vi "MACBIN Create Header__ogtk.vi"(0 "data file":path, 1 "resource file":path, 3 "error in (no error)":errorcluster) -> (4 "comment":string, 5 "header":u8[](array[numeric]), 6 "res size":i32, 7 "data refnum":refnum<file>, 8 "res refnum":refnum<file>, 9 "data size":i32, 10 "error out":errorcluster)   [LabVIEW 2018]
uses:
  <userlib>/_OpenG.lib/lvzip/macbin.llb/MACBIN Macbinary Header__ogtk.ctl
panel:
  in  "macbinary header":T1 {"last mod" format="%<%I:%M:%S %p\n%d/%m/%y>T"; "creation date" format="%<%H:%M:%S\n%d/%m/%y>T"}
  # "Please visit http://www.OpenG.org to learn about the\nOpen Source LabVIEW software movement.\n\nNOTICE -- YOU MUST LEAVE THIS NOTICE IN PLACE.  PER THE TERMS OF THE LICENSE BELOW, YOU MAY SUBLICENSE THIS SOFTWARE \nIN ANY WAY THAT DOES NOT CONFLICT WITH THIS LICENSE.\n\n### BSD License (http://www.opensource.org/licenses/bsd-license.php) Begin ###\n \nCopyright (C) 2002 Christophe Salzmann christophe.salzmann@epfl.ch\nCopyright (C) 2002 Rolf Kalbermatter rolf.kalbermatter@citengineering.com\n\nAll rights reserved.\n\nRedistribution and use in source and binary forms, with or without modification, are permitted provided that the following conditions are met:\n\n    * Redistributions of source code must retain the above copyright notice, this list of conditions and the following disclaimer.\n    * Redistributions in binary form must reproduce the above copyright notice, this list of conditions and the following disclaimer in the \n       documentation and/or other materials provided with the distribution.\n    * Neither the name of SciWare, James Kring, Inc., nor the names of its contributors may be used to endorse or promote products derived \n       from this software without specific prior written permission.\n\nTHIS SOFTWARE IS PROVIDED BY THE COPYRIGHT HOLDERS AND CONTRIBUTORS \"AS IS\" AND ANY EXPRESS OR IMPLIED WARRANTIES, \nINCLUDING, BUT NOT LIMITED TO, THE IMPLIED WARRANTIES OF MERCHANTABILITY AND FITNESS FOR A PARTICULAR PURPOSE ARE \nDISCLAIMED. IN NO EVENT SHALL THE COPYRIGHT OWNER OR CONTRIBUTORS BE LIABLE FOR ANY DIRECT, INDIRECT, INCIDENTAL,\n SPECIAL, EXEMPLARY, OR CONSEQUENTIAL DAMAGES (INCLUDING, BUT NOT LIMITED TO, PROCUREMENT OF SUBSTITUTE GOODS OR \nSERVICES; LOSS OF USE, DATA, OR PROFITS; OR BUSINESS INTERRUPTION) HOWEVER CAUSED AND ON ANY THEORY OF LIABILITY, \nWHETHER IN CONTRACT, STRICT LIABILITY, OR TORT (INCLUDING NEGLIGENCE OR OTHERWISE) ARISING IN ANY WAY OUT OF THE USE \nOF THIS SOFTWARE, EVEN IF ADVISED OF THE POSSIBILITY OF SUCH DAMAGE.\n\n### BSD License End ###"
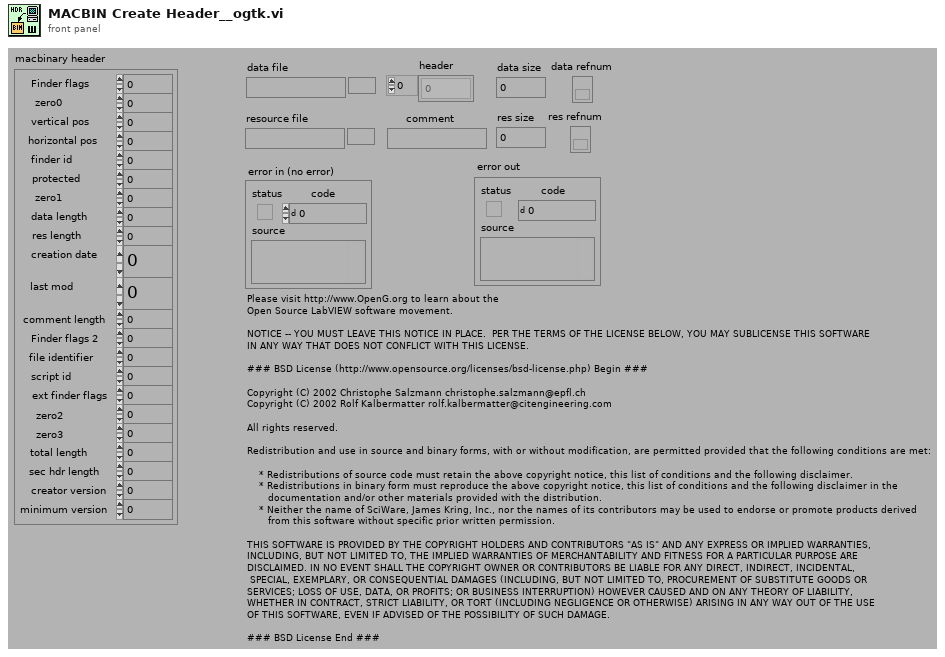
[diagram p1: front panel]
types:
  T1 = typedef "MACBIN Macbinary Header__ogtk.ctl" = cluster{"Finder flags":u8, "zero0":u8, "vertical pos":u16, "horizontal pos":u16, "finder id":u16, "protected":u8, "zero1":u8, "data length":i32, "res length":i32, "creation date":u32, "last mod":u32, "comment length":i16, "Finder flags 2":u8, "file identifier":u32, "script id":u8, "ext finder flags":u8, "zero2":i32, "zero3":i32, "total length":u32, "sec hdr length":u16, "creator version":u8, "minimum version":u8}
  T2 = typedef "MACBIN Resource Header__ogtk.ctl" = cluster{"type":string, "creator":string, "data size":u32, "res size":u32, "creation date":u32, "mod date":u32, "finder flags":u16, "vertical pos":i16, "horizontal pos":i16, "finder id":u16, "script id":u8, "ext finder flags":u8}
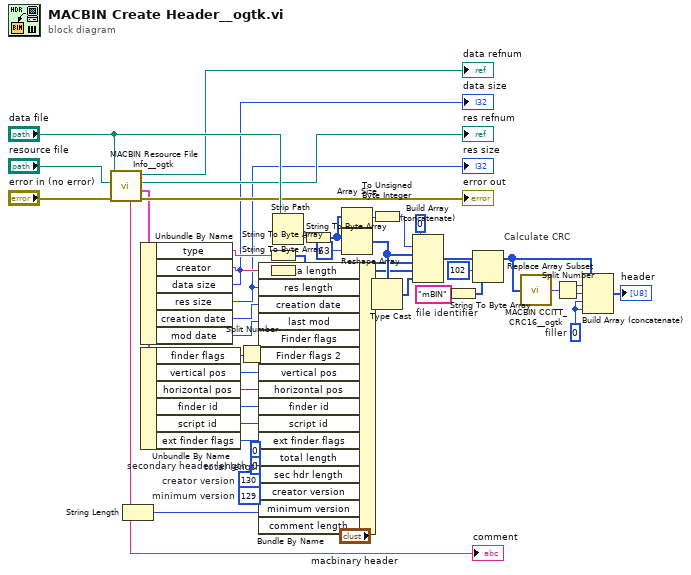
[diagram p0: block diagram]
diagram:
  w38 = u8 0  # filler
  w34 = u32 0  # total length
  w35 = u16 0  # secondary header length
  w36 = u8 130  # creator version
  w37 = u8 129  # minimum version
  w15 = "mBIN"  # file identifier
  # "Calculate CRC"
  n1 = call <userlib>:"MACBIN Resource File Info__ogtk.vi"("error in (no error)"="error in (no error)", "resource file"="resource file", "data file"="data file") -> ("error out"=→"error out":errorcluster, "file info out"=w10:T2, "resource refnum"=→"res refnum":refnum<file>, "data refnum"=→"data refnum":refnum<file>, "comment out"=w26:string)  [unwired: 4 in]
  "comment" <- w26
  n2 = String Length(string=w26) -> (length=w18:i32)
  n3 = Unbundle By Name(w10) -> ("type"=w5:string, "creator"=w9:string, "data size"=w4:u32, "res size"=w3:u32, "creation date"=w25:u32, "mod date"=w19:u32)
  "data size" <- w4
  "res size" <- w3
  n4 = Unbundle By Name(w10) -> ("finder flags"=w11:u16, "vertical pos"=w33:i16, "horizontal pos"=w32:i16, "finder id"=w31:u16, "script id"=w30:u8, "ext finder flags"=w29:u8)
  n5 = Split Number(x=w11) -> (hi(x)=w13:u8, lo(x)=w12:u8)
  n6 = Bundle By Name(cluster="macbinary header", "data length"=w4, "res length"=w3, "creation date"=w25, "last mod"=w19, "Finder flags"=w13, "Finder flags 2"=w12, "vertical pos"=w33, "horizontal pos"=w32, "finder id"=w31, "script id"=w30, "ext finder flags"=w29, "total length"=w34, "sec hdr length"=w35, "creator version"=w36, "minimum version"=w37, "comment length"=w18) -> (w46:T1)
  n7 = String To Byte Array(string=w5) -> (unsigned byte array=w8:u8[])
  n8 = String To Byte Array(string=w9) -> (unsigned byte array=w7:u8[])
  n9 = Strip Path(path="data file") -> (name=w43:string)  [unwired: 1 out]
  n10 = String To Byte Array(string=w43) -> (unsigned byte array=w41:u8[])
  n11 = Array Size(array=w41) -> (size(s)=w42:i32)
  n12 = Reshape Array(w41, 63 ("Dimension Size")) -> (w48:u8[])
  n13 = To Unsigned Byte Integer(number=w42) -> (unsigned 8bit integer=w44:u8)
  n14 = Type Cast(type=w48, x=w46) -> (*(type *) &x=w47:u8[])
  n15 = Build Array (concatenate)(u8 0 ("Input Element"), w44, w48, w8, w7, w47) -> (w17:u8[])
  n16 = String To Byte Array(string=w15) -> (unsigned byte array=w16:u8[])
  n17 = Replace Array Subset(array=w17, new element=w16, index=102 ("Index")) -> (w2:u8[])
  n18 = call <userlib>:"MACBIN CCITT_CRC16__ogtk.vi"("u8 array"=w2) -> ("Checksum"=w1:u16)  [unwired: 4 in]
  n19 = Split Number(x=w1) -> (hi(x)=w20:u8, lo(x)=w21:u8)
  n20 = Build Array (concatenate)(w2, w20, w21, w38, w38) -> (→"header":u8[])
